vi "HandleObservationSync_003.vi"(8 "error in (no error)":errorcluster, 11 "S4GUI in":refnum<class "S4GUI.lvclass">) -> (0 "error out":errorcluster, 3 "S4GUI out":refnum<class "S4GUI.lvclass">)   [LabVIEW 2018, in "S4GUI.lvclass"] (continued)
          n1515 = call-dynamic "Write AcquisitionA.vi"("error in (no error)"=w4306, "Acquisition.lvclass"=w4308, "S4ACS_GUI in"=w4307) -> ("error out"=w4303:errorcluster, "S4ACS_GUI out"=w4302:refnum<class "S4GUI.lvclass">)  [unwired: 7 in]
          n1516 = call "Read AcquisitionB.vi"("error in (no error)"=w4303, "S4ACS_GUI in"=w4302) -> ("error out"=w4281:errorcluster, "Acquisition.lvclass"=w4284:refnum<class "Acquisition.lvclass">, "S4ACS_GUI out"=w4304:refnum<class "S4GUI.lvclass">)  [unwired: 7 in]
          n1517 = call-dynamic "Read enabled.vi"("error in (no error)"=w4281, "Server in"=w4284) -> ("error out"=w4282:errorcluster, "enabled"=w4262:bool, "Server out"=w4283:refnum<class "Acquisition.lvclass">)  [unwired: 7 in]
          n1518 = case shown="True" w4262 {
            tunnel: w4282 -> [w4437 w4454]
            tunnel: w4283 -> [w4438 w4453]
            tunnel: [0 ("State") w4446] -> w4257
            tunnel: [w4437 w4452] -> w4301
            tunnel: [w4438 w4451] -> w4300
            tunnel: w4267 -> [_ w4445]
            tunnel: [TRUE w4444] -> w4268
            tunnel: [FALSE ("stopping") w4440] -> w4253
            frame False {
            }
            frame True {
              n1519 = call-dynamic "Read Channel.vi"("error in (no error)"=w4454, "Acquisition in"=w4453) -> ("error out"=w4449:errorcluster, "Channel.lvclass"=w4450:refnum<class "Channel.lvclass">, "Acquisition out"=w4447:refnum<class "Acquisition.lvclass">)  [unwired: 7 in]
              n1520 = call-dynamic "Read CyclesDone.vi"("error in (no error)"=w4449, "Channel in"=w4450) -> ("error out"=w4442:errorcluster, "CyclesDone"=w4446:u32, "Channel out"=w4448:refnum<class "Channel.lvclass">)  [unwired: 7 in]
              n1521 = Increment(x=w4445) -> (x+1=w4439:u32)
              n1522 = Equal?(x=w4446, y=w4439) -> (x = y?=w4444:bool)
              n1523 = call-dynamic "Read stopping.vi"("error in (no error)"=w4442, "Channel in"=w4448) -> ("error out"=w4441:errorcluster, "stopping"=w4440:bool, "Channel out"=w4443:refnum<class "Channel.lvclass">)  [unwired: 7 in]
              n1524 = call-dynamic "Write Channel.vi"("error in (no error)"=w4441, "Channel.lvclass"=w4443, "Acquisition in"=w4447) -> ("error out"=w4452:errorcluster, "Acquisition out"=w4451:refnum<class "Acquisition.lvclass">)  [unwired: 7 in]
            }
          }
          n1525 = Max & Min(x=w4258, y=w4257) -> (max(x,y)=w4270:u32)  [unwired: 1 out]
          n1526 = call "Write AcquisitionB.vi"("error in (no error)"=w4301, "Acquisition.lvclass"=w4300, "S4ACS_GUI in"=w4304) -> ("error out"=w4293:errorcluster, "S4ACS_GUI out"=w4292:refnum<class "S4GUI.lvclass">)  [unwired: 7 in]
          n1527 = call-dynamic "Read AcquisitionC.vi"("error in (no error)"=w4293, "S4ACS_GUI in"=w4292) -> ("error out"=w4278:errorcluster, "Acquisition.lvclass"=w4280:refnum<class "Acquisition.lvclass">, "S4ACS_GUI out"=w4295:refnum<class "S4GUI.lvclass">)  [unwired: 7 in]
          n1528 = call-dynamic "Read enabled.vi"("error in (no error)"=w4278, "Server in"=w4280) -> ("error out"=w4277:errorcluster, "enabled"=w4261:bool, "Server out"=w4279:refnum<class "Acquisition.lvclass">)  [unwired: 7 in]
          n1529 = case shown="True" w4261 {
            tunnel: [w4416 w4433] -> w4296
            tunnel: [w4417 w4432] -> w4294
            tunnel: w4277 -> [w4416 w4429]
            tunnel: w4279 -> [w4417 w4430]
            tunnel: [0 ("State") w4428] -> w4256
            tunnel: w4267 -> [_ w4427]
            tunnel: [TRUE w4426] -> w4266
            tunnel: [FALSE ("stopping") w4419] -> w4252
            frame False {
            }
            frame True {
              n1530 = call-dynamic "Read Channel.vi"("error in (no error)"=w4429, "Acquisition in"=w4430) -> ("error out"=w4425:errorcluster, "Channel.lvclass"=w4424:refnum<class "Channel.lvclass">, "Acquisition out"=w4431:refnum<class "Acquisition.lvclass">)  [unwired: 7 in]
              n1531 = call-dynamic "Read CyclesDone.vi"("error in (no error)"=w4425, "Channel in"=w4424) -> ("error out"=w4421:errorcluster, "CyclesDone"=w4428:u32, "Channel out"=w4423:refnum<class "Channel.lvclass">)  [unwired: 7 in]
              n1532 = Increment(x=w4427) -> (x+1=w4418:u32)
              n1533 = Equal?(x=w4428, y=w4418) -> (x = y?=w4426:bool)
              n1534 = call-dynamic "Read stopping.vi"("error in (no error)"=w4421, "Channel in"=w4423) -> ("error out"=w4420:errorcluster, "stopping"=w4419:bool, "Channel out"=w4422:refnum<class "Channel.lvclass">)  [unwired: 7 in]
              n1535 = call-dynamic "Write Channel.vi"("error in (no error)"=w4420, "Channel.lvclass"=w4422, "Acquisition in"=w4431) -> ("error out"=w4433:errorcluster, "Acquisition out"=w4432:refnum<class "Acquisition.lvclass">)  [unwired: 7 in]
            }
          }
          n1536 = call-dynamic "Write AcquisitionC.vi"("error in (no error)"=w4296, "Acquisition.lvclass"=w4294, "S4ACS_GUI in"=w4295) -> ("error out"=w4290:errorcluster, "S4ACS_GUI out"=w4291:refnum<class "S4GUI.lvclass">)  [unwired: 7 in]
          n1537 = call-dynamic "Read AcquisitionD.vi"("error in (no error)"=w4290, "S4ACS_GUI in"=w4291) -> ("error out"=w4274:errorcluster, "Acquisition.lvclass"=w4276:refnum<class "Acquisition.lvclass">, "S4ACS_GUI out"=w4297:refnum<class "S4GUI.lvclass">)  [unwired: 7 in]
          n1538 = call-dynamic "Read enabled.vi"("error in (no error)"=w4274, "Server in"=w4276) -> ("error out"=w4273:errorcluster, "enabled"=w4264:bool, "Server out"=w4275:refnum<class "Acquisition.lvclass">)  [unwired: 7 in]
          n1539 = case shown="True" w4264 {
            tunnel: [w4396 w4412] -> w4299
            tunnel: [w4395 w4411] -> w4298
            tunnel: w4275 -> [w4396 w4410]
            tunnel: w4273 -> [w4395 w4409]
            tunnel: [0 ("State") w4407] -> w4255
            tunnel: w4267 -> [_ w4406]
            tunnel: [TRUE w4405] -> w4265
            tunnel: [FALSE ("stopping") w4398] -> w4251
            frame False {
            }
            frame True {
              n1540 = call-dynamic "Read Channel.vi"("error in (no error)"=w4409, "Acquisition in"=w4410) -> ("error out"=w4404:errorcluster, "Channel.lvclass"=w4403:refnum<class "Channel.lvclass">, "Acquisition out"=w4408:refnum<class "Acquisition.lvclass">)  [unwired: 7 in]
              n1541 = call-dynamic "Read CyclesDone.vi"("error in (no error)"=w4404, "Channel in"=w4403) -> ("error out"=w4400:errorcluster, "CyclesDone"=w4407:u32, "Channel out"=w4402:refnum<class "Channel.lvclass">)  [unwired: 7 in]
              n1542 = Increment(x=w4406) -> (x+1=w4397:u32)
              n1543 = Equal?(x=w4407, y=w4397) -> (x = y?=w4405:bool)
              n1544 = call-dynamic "Read stopping.vi"("error in (no error)"=w4400, "Channel in"=w4402) -> ("error out"=w4399:errorcluster, "stopping"=w4398:bool, "Channel out"=w4401:refnum<class "Channel.lvclass">)  [unwired: 7 in]
              n1545 = call-dynamic "Write Channel.vi"("error in (no error)"=w4399, "Channel.lvclass"=w4401, "Acquisition in"=w4408) -> ("error out"=w4411:errorcluster, "Acquisition out"=w4412:refnum<class "Acquisition.lvclass">)  [unwired: 7 in]
            }
          }
          n1546 = Build Array(w4263, w4262, w4261, w4264) -> (w4260:bool[])
          n1547 = Boolean Array To Number(Boolean array=w4260) -> (number=w4259:u32)
          n1548 = Max & Min(x=w4256, y=w4255) -> (max(x,y)=w4269:u32)  [unwired: 1 out]
          n1549 = Compound Arithmetic op=AND(w4271, w4268, w4266, w4265) -> (w4250:bool)
          n1550 = case shown="15" w4259 {
            tunnel: w4258 -> [w4348 _ w4360 _ w4369 _ w4375 w4381 _ w4387 w4390 _]
            tunnel: w4255 -> [w4347 w4351 w4356 w4363 w4364 w4372 w4374 _ _ _ _ _]
            tunnel: w4257 -> [w4346 w4349 _ _ w4368 w4370 _ w4380 w4384 _ w4389 _]
            tunnel: w4256 -> [w4345 w4350 w4355 w4361 _ _ _ w4379 w4383 w4386 _ _]
            tunnel: [w4341 w4352 w4357 w4362 w4365 w4371 w4373 w4376 w4382 w4385 w4388 TRUE] -> _
            frame 15 {
              # "A,B,C,D ativos"
              n1551 = Equal?(x=w4348, y=w4346) -> (x = y?=w4344:bool)
              n1552 = Equal?(x=w4345, y=w4347) -> (x = y?=w4342:bool)
              n1553 = Equal?(x=w4346, y=w4345) -> (x = y?=w4343:bool)
              n1554 = Compound Arithmetic op=AND(w4344, w4343, w4342) -> (w4341:bool)
            }
            frame 14 {
              # "B,C e,D ativos"
              n1555 = Equal?(x=w4349, y=w4350) -> (x = y?=w4354:bool)
              n1556 = Equal?(x=w4350, y=w4351) -> (x = y?=w4353:bool)
              n1557 = Compound Arithmetic op=AND(w4354, w4353) -> (w4352:bool)
            }
            frame 13 {
              # "A,C e,D ativos"
              n1558 = Equal?(x=w4360, y=w4355) -> (x = y?=w4359:bool)
              n1559 = Equal?(x=w4355, y=w4356) -> (x = y?=w4358:bool)
              n1560 = Compound Arithmetic op=AND(w4359, w4358) -> (w4357:bool)
            }
            frame 12 {
              # "Só C e D ativos"
              n1561 = Equal?(x=w4361, y=w4363) -> (x = y?=w4362:bool)
            }
            frame 11 {
              # "A,B e,D ativos"
              n1562 = Equal?(x=w4369, y=w4368) -> (x = y?=w4367:bool)
              n1563 = Equal?(x=w4368, y=w4364) -> (x = y?=w4366:bool)
              n1564 = Compound Arithmetic op=AND(w4367, w4366) -> (w4365:bool)
            }
            frame 10 {
              # "Só B e D ativos"
              n1565 = Equal?(x=w4370, y=w4372) -> (x = y?=w4371:bool)
            }
            frame 9 {
              # "Só A e D ativos"
              n1566 = Equal?(x=w4375, y=w4374) -> (x = y?=w4373:bool)
            }
            frame 7 {
              # "A,B,C ativos"
              n1567 = Equal?(x=w4381, y=w4380) -> (x = y?=w4378:bool)
              n1568 = Equal?(x=w4380, y=w4379) -> (x = y?=w4377:bool)
              n1569 = Compound Arithmetic op=AND(w4378, w4377) -> (w4376:bool)
            }
            frame 6 {
              # "Só B e C ativos"
              n1570 = Equal?(x=w4384, y=w4383) -> (x = y?=w4382:bool)
            }
            frame 5 {
              # "Só A e C ativos"
              n1571 = Equal?(x=w4387, y=w4386) -> (x = y?=w4385:bool)
            }
            frame 3 {
              # "só A e B ativos"
              n1572 = Equal?(x=w4390, y=w4389) -> (x = y?=w4388:bool)
            }
            frame 0..2, 4, 8, Default {
              # "nenhum ou só 1  \ncanal ativo."
            }
          }
          n1573 = Max & Min(x=w4270, y=w4269) -> (max(x,y)=w4248:u32)  [unwired: 1 out]
          n1574 = Compound Arithmetic op=OR(w4254, w4253, w4252, w4251) -> (w4249:bool)
          n1575 = call-dynamic "Write AcquisitionD.vi"("error in (no error)"=w4298, "Acquisition.lvclass"=w4299, "S4ACS_GUI in"=w4297) -> ("error out"=w4289:errorcluster, "S4ACS_GUI out"=w4246:refnum<class "S4GUI.lvclass">)  [unwired: 7 in]
          n1576 = case shown="False" w4250 {
            tunnel: w4246 -> [w4311 w4329]
            tunnel: [w4317 w4328] -> w4245
            tunnel: w4249 -> [_ w4330]
            tunnel: w4248 -> [_ w4327]
            tunnel: w4247 -> [w4309 w4326]
            frame False {
              # "Aguardando iniciar exposição por 5s"
              n1577 = local read "time1"() -> (w4310:u32)
              n1578 = Tick Count (ms)() -> (millisecond timer value=w4316:u32)
              n1579 = Subtract(x=w4316, y=w4310) -> (x-y=w4313:u32)
              n1580 = To Double Precision Float(number=w4313) -> (double precision float=w4315:dbl)
              n1581 = Less?(x=5000.0 ("y"), y=w4315) -> (x < y?=w4314:bool)
              n1582 = case shown="False" w4314 {
                tunnel: w4311 -> [w4321 w4325]
                tunnel: [w4320 w4324] -> w4317
                tunnel: w4309 -> [w4319 _]
                frame False {
                  # "Volta para esperar ACTIVE."
                  n1583 = Decrement(x=w4319) -> (x-1=w4318:u32)
                  n1584 = Bundle By Name(cluster=w4321, "Obs_state"=w4318) -> (w4320:refnum<class "S4GUI.lvclass">)
                }
                frame True {
                  n1585 = Bundle By Name(cluster=w4325, "Obs_state"=u32 1, "Error Msg"="ERROR: Init Acquisition Timeout. HandleObservationSync.vi - state 327.") -> (w4324:refnum<class "S4GUI.lvclass">)
                }
              }
            }
            frame True {
              # "STOP?"
              # "CIclo Avançou."
              n1586 = case shown="False" w4330 {
                tunnel: w4329 -> [w4334 w4340]
                tunnel: [w4333 w4339] -> w4328
                tunnel: w4327 -> [w4332 w4338]
                tunnel: w4326 -> [_ w4337]
                frame True {
                  # "STOP acionado."
                  n1587 = Bundle By Name(cluster=w4334, "Obs_state"=u32 0, "cyclesDone"=w4332) -> (w4333:refnum<class "S4GUI.lvclass">)
                }
                frame False {
                  # "Vai esperar fim da exposição..."
                  n1588 = Increment(x=w4337) -> (x+1=w4336:u32)
                  n1589 = Increment(x=w4336) -> (x+1=w4335:u32)
                  n1590 = Bundle By Name(cluster=w4340, "Obs_state"=w4335, "cyclesDone"=w4338) -> (w4339:refnum<class "S4GUI.lvclass">)
                }
              }
            }
          }
        }
        frame 328 {
          # "T= canais receberam STOP"
          n1591 = Unbundle By Name(w4500) -> ("cyclesDone"=w4494:u32)
          n1592 = call-dynamic "Read AcquisitionA.vi"("error in (no error)"=w4536, "S4ACS_GUI in"=w4500) -> ("error out"=w4515:errorcluster, "Acquisition.lvclass"=w4516:refnum<class "Acquisition.lvclass">, "S4ACS_GUI out"=w4538:refnum<class "S4GUI.lvclass">)  [unwired: 7 in]
          n1593 = call-dynamic "Read enabled.vi"("error in (no error)"=w4515, "Server in"=w4516) -> ("error out"=w4514:errorcluster, "enabled"=w4490:bool, "Server out"=w4513:refnum<class "Acquisition.lvclass">)  [unwired: 7 in]
          n1594 = case shown="True" w4490 {
            tunnel: w4514 -> [w4687 w4704]
            tunnel: [w4688 w4702] -> w4539
            tunnel: [w4687 w4701] -> w4537
            tunnel: [0 ("State") w4697] -> w4485
            tunnel: w4513 -> [w4688 w4696]
            tunnel: w4494 -> [_ w4695]
            tunnel: [TRUE w4694] -> w4499
            tunnel: [FALSE ("stopping") w4690] -> w4481
            frame False {
            }
            frame True {
              n1595 = call-dynamic "Read Channel.vi"("error in (no error)"=w4704, "Acquisition in"=w4696) -> ("error out"=w4700:errorcluster, "Channel.lvclass"=w4699:refnum<class "Channel.lvclass">, "Acquisition out"=w4703:refnum<class "Acquisition.lvclass">)  [unwired: 7 in]
              n1596 = call-dynamic "Read CyclesDone.vi"("error in (no error)"=w4700, "Channel in"=w4699) -> ("error out"=w4692:errorcluster, "CyclesDone"=w4697:u32, "Channel out"=w4698:refnum<class "Channel.lvclass">)  [unwired: 7 in]
              n1597 = Increment(x=w4695) -> (x+1=w4689:u32)
              n1598 = Equal?(x=w4697, y=w4689) -> (x = y?=w4694:bool)
              n1599 = call-dynamic "Read stopping.vi"("error in (no error)"=w4692, "Channel in"=w4698) -> ("error out"=w4691:errorcluster, "stopping"=w4690:bool, "Channel out"=w4693:refnum<class "Channel.lvclass">)  [unwired: 7 in]
              n1600 = call-dynamic "Write Channel.vi"("error in (no error)"=w4691, "Channel.lvclass"=w4693, "Acquisition in"=w4703) -> ("error out"=w4701:errorcluster, "Acquisition out"=w4702:refnum<class "Acquisition.lvclass">)  [unwired: 7 in]
            }
          }
          n1601 = call-dynamic "Write AcquisitionA.vi"("error in (no error)"=w4537, "Acquisition.lvclass"=w4539, "S4ACS_GUI in"=w4538) -> ("error out"=w4532:errorcluster, "S4ACS_GUI out"=w4531:refnum<class "S4GUI.lvclass">)  [unwired: 7 in]
          n1602 = call "Read AcquisitionB.vi"("error in (no error)"=w4532, "S4ACS_GUI in"=w4531) -> ("error out"=w4509:errorcluster, "Acquisition.lvclass"=w4512:refnum<class "Acquisition.lvclass">, "S4ACS_GUI out"=w4533:refnum<class "S4GUI.lvclass">)  [unwired: 7 in]
          n1603 = call-dynamic "Read enabled.vi"("error in (no error)"=w4509, "Server in"=w4512) -> ("error out"=w4510:errorcluster, "enabled"=w4489:bool, "Server out"=w4511:refnum<class "Acquisition.lvclass">)  [unwired: 7 in]
          n1604 = case shown="True" w4489 {
            tunnel: w4510 -> [w4666 w4683]
            tunnel: w4511 -> [w4667 w4682]
            tunnel: [0 ("State") w4675] -> w4484
            tunnel: [w4666 w4681] -> w4530
            tunnel: [w4667 w4680] -> w4529
            tunnel: w4494 -> [_ w4674]
            tunnel: [TRUE w4673] -> w4495
            tunnel: [FALSE ("stopping") w4669] -> w4480
            frame False {
            }
            frame True {
              n1605 = call-dynamic "Read Channel.vi"("error in (no error)"=w4683, "Acquisition in"=w4682) -> ("error out"=w4678:errorcluster, "Channel.lvclass"=w4679:refnum<class "Channel.lvclass">, "Acquisition out"=w4676:refnum<class "Acquisition.lvclass">)  [unwired: 7 in]
              n1606 = call-dynamic "Read CyclesDone.vi"("error in (no error)"=w4678, "Channel in"=w4679) -> ("error out"=w4671:errorcluster, "CyclesDone"=w4675:u32, "Channel out"=w4677:refnum<class "Channel.lvclass">)  [unwired: 7 in]
              n1607 = Increment(x=w4674) -> (x+1=w4668:u32)
              n1608 = Equal?(x=w4675, y=w4668) -> (x = y?=w4673:bool)
              n1609 = call-dynamic "Read stopping.vi"("error in (no error)"=w4671, "Channel in"=w4677) -> ("error out"=w4670:errorcluster, "stopping"=w4669:bool, "Channel out"=w4672:refnum<class "Channel.lvclass">)  [unwired: 7 in]
              n1610 = call-dynamic "Write Channel.vi"("error in (no error)"=w4670, "Channel.lvclass"=w4672, "Acquisition in"=w4676) -> ("error out"=w4681:errorcluster, "Acquisition out"=w4680:refnum<class "Acquisition.lvclass">)  [unwired: 7 in]
            }
          }
          n1611 = Max & Min(x=w4485, y=w4484) -> (max(x,y)=w4498:u32)  [unwired: 1 out]
          n1612 = call "Write AcquisitionB.vi"("error in (no error)"=w4530, "Acquisition.lvclass"=w4529, "S4ACS_GUI in"=w4533) -> ("error out"=w4522:errorcluster, "S4ACS_GUI out"=w4521:refnum<class "S4GUI.lvclass">)  [unwired: 7 in]
          n1613 = call-dynamic "Read AcquisitionC.vi"("error in (no error)"=w4522, "S4ACS_GUI in"=w4521) -> ("error out"=w4506:errorcluster, "Acquisition.lvclass"=w4508:refnum<class "Acquisition.lvclass">, "S4ACS_GUI out"=w4524:refnum<class "S4GUI.lvclass">)  [unwired: 7 in]
          n1614 = call-dynamic "Read enabled.vi"("error in (no error)"=w4506, "Server in"=w4508) -> ("error out"=w4505:errorcluster, "enabled"=w4488:bool, "Server out"=w4507:refnum<class "Acquisition.lvclass">)  [unwired: 7 in]
          n1615 = case shown="True" w4488 {
            tunnel: [w4645 w4662] -> w4525
            tunnel: [w4646 w4661] -> w4523
            tunnel: w4505 -> [w4645 w4658]
            tunnel: w4507 -> [w4646 w4659]
            tunnel: [0 ("State") w4657] -> w4483
            tunnel: w4494 -> [_ w4656]
            tunnel: [TRUE w4655] -> w4493
            tunnel: [FALSE ("stopping") w4648] -> w4479
            frame False {
            }
            frame True {
              n1616 = call-dynamic "Read Channel.vi"("error in (no error)"=w4658, "Acquisition in"=w4659) -> ("error out"=w4654:errorcluster, "Channel.lvclass"=w4653:refnum<class "Channel.lvclass">, "Acquisition out"=w4660:refnum<class "Acquisition.lvclass">)  [unwired: 7 in]
              n1617 = call-dynamic "Read CyclesDone.vi"("error in (no error)"=w4654, "Channel in"=w4653) -> ("error out"=w4650:errorcluster, "CyclesDone"=w4657:u32, "Channel out"=w4652:refnum<class "Channel.lvclass">)  [unwired: 7 in]
              n1618 = Increment(x=w4656) -> (x+1=w4647:u32)
              n1619 = Equal?(x=w4657, y=w4647) -> (x = y?=w4655:bool)
              n1620 = call-dynamic "Read stopping.vi"("error in (no error)"=w4650, "Channel in"=w4652) -> ("error out"=w4649:errorcluster, "stopping"=w4648:bool, "Channel out"=w4651:refnum<class "Channel.lvclass">)  [unwired: 7 in]
              n1621 = call-dynamic "Write Channel.vi"("error in (no error)"=w4649, "Channel.lvclass"=w4651, "Acquisition in"=w4660) -> ("error out"=w4662:errorcluster, "Acquisition out"=w4661:refnum<class "Acquisition.lvclass">)  [unwired: 7 in]
            }
          }
          n1622 = call-dynamic "Write AcquisitionC.vi"("error in (no error)"=w4525, "Acquisition.lvclass"=w4523, "S4ACS_GUI in"=w4524) -> ("error out"=w4519:errorcluster, "S4ACS_GUI out"=w4520:refnum<class "S4GUI.lvclass">)  [unwired: 7 in]
          n1623 = call-dynamic "Read AcquisitionD.vi"("error in (no error)"=w4519, "S4ACS_GUI in"=w4520) -> ("error out"=w4502:errorcluster, "Acquisition.lvclass"=w4504:refnum<class "Acquisition.lvclass">, "S4ACS_GUI out"=w4526:refnum<class "S4GUI.lvclass">)  [unwired: 7 in]
          n1624 = call-dynamic "Read enabled.vi"("error in (no error)"=w4502, "Server in"=w4504) -> ("error out"=w4501:errorcluster, "enabled"=w4491:bool, "Server out"=w4503:refnum<class "Acquisition.lvclass">)  [unwired: 7 in]
          n1625 = case shown="True" w4491 {
            tunnel: [w4625 w4641] -> w4528
            tunnel: [w4624 w4640] -> w4527
            tunnel: w4503 -> [w4625 w4639]
            tunnel: w4501 -> [w4624 w4638]
            tunnel: [0 ("State") w4636] -> w4482
            tunnel: w4494 -> [_ w4635]
            tunnel: [TRUE w4634] -> w4492
            tunnel: [FALSE ("stopping") w4627] -> w4478
            frame False {
            }
            frame True {
              n1626 = call-dynamic "Read Channel.vi"("error in (no error)"=w4638, "Acquisition in"=w4639) -> ("error out"=w4633:errorcluster, "Channel.lvclass"=w4632:refnum<class "Channel.lvclass">, "Acquisition out"=w4637:refnum<class "Acquisition.lvclass">)  [unwired: 7 in]
              n1627 = call-dynamic "Read CyclesDone.vi"("error in (no error)"=w4633, "Channel in"=w4632) -> ("error out"=w4629:errorcluster, "CyclesDone"=w4636:u32, "Channel out"=w4631:refnum<class "Channel.lvclass">)  [unwired: 7 in]
              n1628 = Increment(x=w4635) -> (x+1=w4626:u32)
              n1629 = Equal?(x=w4636, y=w4626) -> (x = y?=w4634:bool)
              n1630 = call-dynamic "Read stopping.vi"("error in (no error)"=w4629, "Channel in"=w4631) -> ("error out"=w4628:errorcluster, "stopping"=w4627:bool, "Channel out"=w4630:refnum<class "Channel.lvclass">)  [unwired: 7 in]
              n1631 = call-dynamic "Write Channel.vi"("error in (no error)"=w4628, "Channel.lvclass"=w4630, "Acquisition in"=w4637) -> ("error out"=w4640:errorcluster, "Acquisition out"=w4641:refnum<class "Acquisition.lvclass">)  [unwired: 7 in]
            }
          }
          n1632 = Build Array(w4490, w4489, w4488, w4491) -> (w4487:bool[])
          n1633 = Boolean Array To Number(Boolean array=w4487) -> (number=w4486:u32)
          n1634 = Max & Min(x=w4483, y=w4482) -> (max(x,y)=w4497:u32)  [unwired: 1 out]
          n1635 = Compound Arithmetic op=AND(w4499, w4495, w4493, w4492) -> (w4476:bool)
          n1636 = case shown="15" w4486 {
            tunnel: w4485 -> [w4547 _ w4559 _ w4568 _ w4574 w4580 _ w4586 w4589 _]
            tunnel: w4482 -> [w4546 w4550 w4555 w4562 w4563 w4571 w4573 _ _ _ _ _]
            tunnel: w4484 -> [w4545 w4548 _ _ w4567 w4569 _ w4579 w4583 _ w4588 _]
            tunnel: w4483 -> [w4544 w4549 w4554 w4560 _ _ _ w4578 w4582 w4585 _ _]
            tunnel: [w4540 w4551 w4556 w4561 w4564 w4570 w4572 w4575 w4581 w4584 w4587 TRUE] -> _
            frame 15 {
              # "A,B,C,D ativos"
              n1637 = Equal?(x=w4547, y=w4545) -> (x = y?=w4543:bool)
              n1638 = Equal?(x=w4544, y=w4546) -> (x = y?=w4541:bool)
              n1639 = Equal?(x=w4545, y=w4544) -> (x = y?=w4542:bool)
              n1640 = Compound Arithmetic op=AND(w4543, w4542, w4541) -> (w4540:bool)
            }
            frame 14 {
              # "B,C e,D ativos"
              n1641 = Equal?(x=w4548, y=w4549) -> (x = y?=w4553:bool)
              n1642 = Equal?(x=w4549, y=w4550) -> (x = y?=w4552:bool)
              n1643 = Compound Arithmetic op=AND(w4553, w4552) -> (w4551:bool)
            }
            frame 13 {
              # "A,C e,D ativos"
              n1644 = Equal?(x=w4559, y=w4554) -> (x = y?=w4558:bool)
              n1645 = Equal?(x=w4554, y=w4555) -> (x = y?=w4557:bool)
              n1646 = Compound Arithmetic op=AND(w4558, w4557) -> (w4556:bool)
            }
            frame 12 {
              # "Só C e D ativos"
              n1647 = Equal?(x=w4560, y=w4562) -> (x = y?=w4561:bool)
            }
            frame 11 {
              # "A,B e,D ativos"
              n1648 = Equal?(x=w4568, y=w4567) -> (x = y?=w4566:bool)
              n1649 = Equal?(x=w4567, y=w4563) -> (x = y?=w4565:bool)
              n1650 = Compound Arithmetic op=AND(w4566, w4565) -> (w4564:bool)
            }
            frame 10 {
              # "Só B e D ativos"
              n1651 = Equal?(x=w4569, y=w4571) -> (x = y?=w4570:bool)
            }
            frame 9 {
              # "Só A e D ativos"
              n1652 = Equal?(x=w4574, y=w4573) -> (x = y?=w4572:bool)
            }
            frame 7 {
              # "A,B,C ativos"
              n1653 = Equal?(x=w4580, y=w4579) -> (x = y?=w4577:bool)
              n1654 = Equal?(x=w4579, y=w4578) -> (x = y?=w4576:bool)
              n1655 = Compound Arithmetic op=AND(w4577, w4576) -> (w4575:bool)
            }
            frame 6 {
              # "Só B e C ativos"
              n1656 = Equal?(x=w4583, y=w4582) -> (x = y?=w4581:bool)
            }
            frame 5 {
              # "Só A e C ativos"
              n1657 = Equal?(x=w4586, y=w4585) -> (x = y?=w4584:bool)
            }
            frame 3 {
              # "só A e B ativos"
              n1658 = Equal?(x=w4589, y=w4588) -> (x = y?=w4587:bool)
            }
            frame 0..2, 4, 8, Default {
              # "nenhum ou só 1  \ncanal ativo."
            }
          }
          n1659 = Max & Min(x=w4498, y=w4497) -> (max(x,y)=w4496:u32)  [unwired: 1 out]
          n1660 = Compound Arithmetic op=OR(w4481, w4480, w4479, w4478) -> (w4477:bool)
          n1661 = call-dynamic "Write AcquisitionD.vi"("error in (no error)"=w4527, "Acquisition.lvclass"=w4528, "S4ACS_GUI in"=w4526) -> ("error out"=w4517:errorcluster, "S4ACS_GUI out"=w4518:refnum<class "S4GUI.lvclass">)  [unwired: 7 in]
          n1662 = case shown="True" w4476 {
            tunnel: w4518 -> [w4601 w4611]
            tunnel: [w4600 w4610] -> w4535
            tunnel: w4534 -> [_ w4609]
            tunnel: w4496 -> [_ w4608]
            tunnel: w4477 -> [_ w4607]
            frame False {
              # "Aguardando avanço do ciclo."
              n1663 = local read "time307"() -> (w4591:u32)
              n1664 = Tick Count (ms)() -> (millisecond timer value=w4599:u32)
              n1665 = Subtract(x=w4599, y=w4591) -> (x-y=w4596:u32)
              n1666 = call-dynamic "GetGreatestCube.vi"("S4GUI in"=w4601) -> ("S4GUI out"=w4592:refnum<class "S4GUI.lvclass">, "greatest (ms)"=w4594:dbl)  [unwired: 8 in, 1 out]
              n1667 = To Double Precision Float(number=w4596) -> (double precision float=w4598:dbl)
              n1668 = Add(x=5000.0 ("y"), y=w4594) -> (x+y=w4593:dbl)
              n1669 = Less?(x=w4593, y=w4598) -> (x < y?=w4597:bool)
              n1670 = case shown="True" w4597 {
                tunnel: w4592 -> [w4602 w4606]
                tunnel: [w4602 w4605] -> w4600
                frame False {
                }
                frame True {
                  n1671 = Bundle By Name(cluster=w4606, "Obs_state"=u32 1, "Error Msg"="ERROR: Acquisition Timeout. HandleObservationSync.vi - state 328.") -> (w4605:refnum<class "S4GUI.lvclass">)
                }
              }
            }
            frame True {
              # "Ciclo avançou."
              # "STOP?"
              n1672 = case shown="False" w4607 {
                tunnel: w4611 -> [w4615 w4620]
                tunnel: [w4614 w4619] -> w4610
                tunnel: w4609 -> [_ w4617]
                tunnel: w4608 -> [w4613 w4616]
                frame True {
                  n1673 = Bundle By Name(cluster=w4615, "Obs_state"=u32 0, "cyclesDone"=w4613) -> (w4614:refnum<class "S4GUI.lvclass">)
                }
                frame False {
                  n1674 = Increment(x=w4617) -> (x+1=w4618:u32)
                  n1675 = Bundle By Name(cluster=w4620, "Obs_state"=w4618, "cyclesDone"=w4616) -> (w4619:refnum<class "S4GUI.lvclass">)
                }
              }
            }
          }
        }
        frame 329 {
          n1676 = disable-structure shown="Enabled" {
            disable-tunnel: w4709 -> [w4723 w4729]
            disable-tunnel: w4708 -> [w4722 w4736]
            disable-tunnel: [w4721 w4736] -> w4707
            disable-tunnel: [w4719 w4737] -> w4706
            disable-tunnel: w4705 -> [_ w4730]
            frame Disabled {
              n1677 = call-dynamic "Read ciclos.vi"("error in (no error)"=w4722, "S4ACS_GUI in"=w4723) -> ("error out"=w4711:errorcluster, "ciclos"=w4716:u32, "S4ACS_GUI out"=w4724:refnum<class "S4GUI.lvclass">)  [unwired: 7 in]
              n1678 = Decrement(x=w4716) -> (x-1=w4710:u32)
              n1679 = Greater Than 0?(x=w4710) -> (x > 0?=w4717:bool)
              n1680 = case shown="False" w4717 {
                selector: w4717 -> [w4726 w4728]
                tunnel: w4710 -> [_ w4727]
                tunnel: [w4726 w4728] -> w4715
                tunnel: [u32 0 w4727] -> w4712
                frame False {
                }
                frame True {
                }
              }
              n1681 = Select(t=u32 323, s=w4715, f=u32 0) -> (s? t:f=w4718:u32)
              n1682 = call-dynamic "Write ciclos.vi"("error in (no error)"=w4711, "ciclos"=w4712, "S4ACS_GUI in"=w4724) -> ("error out"=w4721:errorcluster, "S4ACS_GUI out"=w4720:refnum<class "S4GUI.lvclass">)  [unwired: 7 in]
              n1683 = Bundle By Name(cluster=w4720, "Obs_state"=w4718) -> (w4719:refnum<class "S4GUI.lvclass">)
            }
            frame Enabled {
              n1684 = Unbundle By Name(w4729) -> ("TotalCiclos"=w4739:u32, "cyclesDone"=w4738:u32)
              n1685 = Subtract(x=w4739, y=w4738) -> (x-y=w4732:u32)
              n1686 = Greater Than 0?(x=w4732) -> (x > 0?=w4735:bool)
              n1687 = disable-structure shown="Enabled" {
                disable-tunnel: [w4741 u32 325 ("t")] -> w4731
                disable-tunnel: w4730 -> [w4740 _]
                frame Disabled {
                  n1688 = Increment(x=w4740) -> (x+1=w4741:u32)
                }
                frame Enabled {
                }
              }
              n1689 = Select(t=w4731, s=w4735, f=u32 0) -> (s? t:f=w4734:u32)
              n1690 = Bundle By Name(cluster=w4729, "ciclos"=w4732, "Obs_state"=w4734) -> (w4737:refnum<class "S4GUI.lvclass">)
            }
          }
        }
        frame 350 {
          n1691 = flat-sequence {
            tunnel: w4744 -> [w4784]
            tunnel: [w4784] -> w4743
            frame #0 {
              n1692 = Tick Count (ms)() -> (millisecond timer value=→"timer350":u32)
            }
          }
          n1693 = call "Read Instrument.lvclass.vi"("error in (no error)"=w4743, "S4ACS_GUI in"=w4779) -> ("error out"=w4782:errorcluster, "Instrument.lvclass"=w4783:refnum<class "Instrument.lvclass">, "S4ACS_GUI out"=w4780:refnum<class "S4GUI.lvclass">)  [unwired: 7 in]
          n1694 = call "Read WPROT.vi"("error in (no error)"=w4782, "Instrument in"=w4783) -> ("error out"=w4772:errorcluster, "Opt_Selector.lvclass"=w4773:refnum<class "Opt_Selector.lvclass">, "Instrument out"=w4781:refnum<class "Instrument.lvclass">)  [unwired: 7 in]
          n1695 = call-dynamic "getTargetPos.vi"("error in (no error)"=w4772, "Opt_Selector in"=w4773) -> ("error out"=w4771:errorcluster, "Target Pos"=w4751:u16, "Opt_Selector out"=w4770:refnum<class "Opt_Selector.lvclass">)  [unwired: 7 in]
          n1696 = Build Array(-1.0 ("element"), 0.0 ("element"), 22.5 ("element"), 45.0 ("element"), 67.5 ("element"), 90.0 ("element"), 112.5 ("element"), 135.0 ("element"), 157.5 ("element"), 180.0 ("element"), 202.5 ("element"), 225.0 ("element"), 247.5 ("element"), 270.0 ("element"), 292.5 ("element"), 315.0 ("element"), 337.5 ("element")) -> (w4763:dbl[])
          n1697 = Index Array(array=w4763, index=w4751) -> (element=w4750:dbl)
          n1698 = case shown="0, Default" w4751 {
            selector: w4751 -> [_ w4813]
            tunnel: w4781 -> [w4793 w4801]
            tunnel: [w4793 w4801] -> w4746
            tunnel: [w4790 w4800] -> w4745
            tunnel: w4776 -> [_ w4815]
            tunnel: [u32 352 w4814] -> w4775
            tunnel: w4771 -> [w4791 w4809]
            tunnel: w4770 -> [w4792 w4808]
            tunnel: w4750 -> [_ w4803]
            tunnel: [w4788 w4802] -> w4747
            frame 0, Default {
              # "Terminou uma sequência.\nRecupera as posições em SEQ e desvia para 311 para verificar se há mais ciclos."
              # "Recupera a sequencia anterior para o caso \nde repetição da sequencia (sem precisar clicar \nnas posicoes desejadas novamente)."
              n1699 = call-dynamic "Read sequencia_ant.vi"("error in (no error)"=w4791, "Opt_Selector in"=w4792) -> ("error out"=w4787:errorcluster, "sequencia_ant"=w4786:u16, "Opt_Selector out"=w4789:refnum<class "Opt_Selector.lvclass">)  [unwired: 7 in]
              n1700 = call-dynamic "Write sequencia.vi"("error in (no error)"=w4787, "sequencia"=w4786, "Opt_Selector in"=w4789) -> ("error out"=w4790:errorcluster, "Opt_Selector out"=w4788:refnum<class "Opt_Selector.lvclass">)  [unwired: 7 in]
            }
            frame 1..16 {
              # "Espera até 40 x 0.25s (= 10s) para\nmecanismo entrar em READY"
              n1701 = Number To Decimal String(number=w4813) -> (decimal integer string=w4812:string)  [unwired: 1 in]
              n1702 = Concatenate Strings("WP" ("string"), w4812) -> (w4810:string)
              n1703 = call "Write target name.vi"("error in (no error)"=w4809, "target name"=w4810, "Optics in"=w4808) -> ("error out"=w4806:errorcluster, "Optics out"=w4807:refnum<class "Opt_Selector.lvclass">)  [unwired: 7 in]
              n1704 = call "Write target.vi"("error in (no error)"=w4806, "target"=w4803, "Optics in"=w4807) -> ("error out"=w4805:errorcluster, "Optics out"=w4804:refnum<class "Opt_Selector.lvclass">)  [unwired: 7 in]
              n1705 = call-dynamic "Read State Machine.vi"("error in (no error)"=w4805, "Device in"=w4804) -> ("error out"=w4817:errorcluster, "State Machine.lvclass"=w4819:refnum<class "State Machine.lvclass">, "Device out"=w4816:refnum<class "Opt_Selector.lvclass">)  [unwired: 7 in]
              n1706 = Increment(x=w4815) -> (x+1=w4814:u32)
              n1707 = call "Next State.vi"("error in (no error)"=w4817, "New_State"=1, "State Machine in"=w4819) -> ("error out"=w4797:errorcluster, "State Machine out"=w4799:refnum<class "State Machine.lvclass">)  [unwired: 7 in]
              n1708 = call-dynamic "Write Timer.vi"("error in (no error)"=w4797, "Timer"=u32 40, "State Machine in"=w4799) -> ("error out"=w4796:errorcluster, "State Machine out"=w4798:refnum<class "State Machine.lvclass">)  [unwired: 7 in]
              n1709 = call-dynamic "Write State Machine.vi"("error in (no error)"=w4796, "State Machine.lvclass"=w4798, "Device in"=w4816) -> ("error out"=w4800:errorcluster, "Device out"=w4802:refnum<class "Opt_Selector.lvclass">)  [unwired: 7 in]
            }
          }
          n1710 = call "Write WPROT.vi"("error in (no error)"=w4745, "Opt_Selector.lvclass"=w4747, "Instrument in"=w4746) -> ("error out"=w4749:errorcluster, "Instrument out"=w4748:refnum<class "Instrument.lvclass">)  [unwired: 7 in]
          n1711 = call "Write Instrument.lvclass.vi"("error in (no error)"=w4749, "Instrument.lvclass"=w4748, "S4ACS_GUI in"=w4780) -> ("error out"=w4778:errorcluster, "S4ACS_GUI out"=w4777:refnum<class "S4GUI.lvclass">)  [unwired: 7 in]
          n1712 = Bundle By Name(cluster=w4777, "Obs_state"=w4775) -> (w4774:refnum<class "S4GUI.lvclass">)
        }
        frame 351 {
          # "Espera terminar o movimento da lamina para disparar a aquisição\ndos canais ativos.\n\nOV 20230424: Não precisa mais atualizar o valor de WPPOS com o\ncomando WRITE_HEADER porque o ACS já recebeu a sequência de\nposições da lâmina."
          n1713 = flat-sequence {
            tunnel: w4830 -> [w4849]
            tunnel: [w4849] -> w4829
            frame #0 {
              n1714 = Tick Count (ms)() -> (millisecond timer value=w4848:u32)
              "timer351" <- w4848
              n1715 = local read "time1"() -> (w4847:u32)
              n1716 = Subtract(x=w4848, y=w4847) -> (x-y=→"delay wp 2":u32)
            }
          }
          n1717 = call "Read Instrument.lvclass.vi"("error in (no error)"=w4829, "S4ACS_GUI in"=w4839) -> ("error out"=w4844:errorcluster, "Instrument.lvclass"=w4845:refnum<class "Instrument.lvclass">, "S4ACS_GUI out"=w4841:refnum<class "S4GUI.lvclass">)  [unwired: 7 in]
          n1718 = call "Read WPROT.vi"("error in (no error)"=w4844, "Instrument in"=w4845) -> ("error out"=w4836:errorcluster, "Opt_Selector.lvclass"=w4835:refnum<class "Opt_Selector.lvclass">, "Instrument out"=w4843:refnum<class "Instrument.lvclass">)  [unwired: 7 in]
          n1719 = call-dynamic "Read State Machine.vi"("error in (no error)"=w4836, "Device in"=w4835) -> ("error out"=w4837:errorcluster, "State Machine.lvclass"=w4838:refnum<class "State Machine.lvclass">, "Device out"=w4833:refnum<class "Opt_Selector.lvclass">)  [unwired: 7 in]
          n1720 = call-dynamic "Read State.vi"("error in (no error)"=w4837, "State Machine in"=w4838) -> ("error out"=w4827:errorcluster, "State"=w4831:i32, "State Machine out"=w4828:refnum<class "State Machine.lvclass">)  [unwired: 7 in]
          n1721 = Equal To 0?(x=w4831) -> (x = 0?=w4822:bool)
          n1722 = call-dynamic "Write State Machine.vi"("error in (no error)"=w4827, "State Machine.lvclass"=w4828, "Device in"=w4833) -> ("error out"=w4832:errorcluster, "Device out"=w4834:refnum<class "Opt_Selector.lvclass">)  [unwired: 7 in]
          n1723 = call "Write WPROT.vi"("error in (no error)"=w4832, "Opt_Selector.lvclass"=w4834, "Instrument in"=w4843) -> ("error out"=w4840:errorcluster, "Instrument out"=w4842:refnum<class "Instrument.lvclass">)  [unwired: 7 in]
          n1724 = call "Write Instrument.lvclass.vi"("error in (no error)"=w4840, "Instrument.lvclass"=w4842, "S4ACS_GUI in"=w4841) -> ("error out"=w4820:errorcluster, "S4ACS_GUI out"=w4823:refnum<class "S4GUI.lvclass">)  [unwired: 7 in]
          n1725 = Select(t=u32 350, s=w4822, f=w4821) -> (s? t:f=w4826:u32)
          n1726 = Bundle By Name(cluster=w4823, "Obs_state"=w4826) -> (w4824:refnum<class "S4GUI.lvclass">)
        }
        frame 352 {
          n1727 = disable-structure shown="Enabled" {
            disable-tunnel: w4853 -> [w4867 w4880]
            disable-tunnel: w4852 -> [w4866 w4878]
            disable-tunnel: [w4865 w4878] -> w4851
            disable-tunnel: [w4863 w4879] -> w4850
            frame Disabled {
              n1728 = call-dynamic "Read ciclos.vi"("error in (no error)"=w4866, "S4ACS_GUI in"=w4867) -> ("error out"=w4855:errorcluster, "ciclos"=w4860:u32, "S4ACS_GUI out"=w4868:refnum<class "S4GUI.lvclass">)  [unwired: 7 in]
              n1729 = Decrement(x=w4860) -> (x-1=w4854:u32)
              n1730 = Greater Than 0?(x=w4854) -> (x > 0?=w4861:bool)
              n1731 = case shown="False" w4861 {
                selector: w4861 -> [w4870 w4872]
                tunnel: w4854 -> [_ w4871]
                tunnel: [w4870 w4872] -> w4859
                tunnel: [u32 0 w4871] -> w4856
                frame False {
                }
                frame True {
                }
              }
              n1732 = Select(t=u32 323, s=w4859, f=u32 0) -> (s? t:f=w4862:u32)
              n1733 = call-dynamic "Write ciclos.vi"("error in (no error)"=w4855, "ciclos"=w4856, "S4ACS_GUI in"=w4868) -> ("error out"=w4865:errorcluster, "S4ACS_GUI out"=w4864:refnum<class "S4GUI.lvclass">)  [unwired: 7 in]
              n1734 = Bundle By Name(cluster=w4864, "Obs_state"=w4862) -> (w4863:refnum<class "S4GUI.lvclass">)
            }
            frame Enabled {
              n1735 = Unbundle By Name(w4880) -> ("cycles wprot"=w4881:u32)
              n1736 = Decrement(x=w4881) -> (x-1=w4873:u32)
              n1737 = Greater Than 0?(x=w4873) -> (x > 0?=w4877:bool)
              n1738 = Select(t=u32 350, s=w4877, f=u32 0) -> (s? t:f=w4876:u32)
              n1739 = Bundle By Name(cluster=w4880, "Obs_state"=w4876, "cycles wprot"=w4873) -> (w4879:refnum<class "S4GUI.lvclass">)
            }
          }
        }
        frame 360 {
          w4882 = u32 0 ("cyclesDone")
          # "Inicia o Ticks com\nvalor do relogio atual"
          # "Espera até 40 x 0.25s (= 10s) para\nmecanismo entrar em READY"
          # "Busca próximo valor de foco..."
          n1740 = flat-sequence {
            tunnel: w4899 -> [w4914]
            tunnel: [w4914] -> w4898
            frame #0 {
              n1741 = Tick Count (ms)() -> (millisecond timer value=→"time7":u32)
            }
          }
          n1742 = call-dynamic "Read TelFocus.lvclass.vi"("error in (no error)"=w4898, "S4GUI in"=w4910) -> ("error out"=w4912:errorcluster, "TelFocus.lvclass"=w4913:refnum<class "TelFocus.lvclass">, "S4GUI out"=w4911:refnum<class "S4GUI.lvclass">)  [unwired: 7 in]
          n1743 = call-dynamic "GetNextFocus.vi"("error in (no error)"=w4912, "TelFocus in"=w4913) -> ("error out"=w4896:errorcluster, "TelFocus out"=w4897:refnum<class "TelFocus.lvclass">)  [unwired: 8 in]
          n1744 = call-dynamic "Read SecMirror.lvclass.vi"("error in (no error)"=w4896, "TelFocus in"=w4897) -> ("error out"=w4883:errorcluster, "SecMirror.lvclass"=w4884:refnum<class "SecMirror.lvclass">, "TelFocus out"=w4901:refnum<class "TelFocus.lvclass">)  [unwired: 7 in]
          n1745 = call-dynamic "Read State Machine.vi"("error in (no error)"=w4883, "Device in"=w4884) -> ("error out"=w4893:errorcluster, "State Machine.lvclass"=w4895:refnum<class "State Machine.lvclass">, "Device out"=w4892:refnum<class "SecMirror.lvclass">)  [unwired: 7 in]
          n1746 = call "Next State.vi"("error in (no error)"=w4893, "New_State"=1, "State Machine in"=w4895) -> ("error out"=w4890:errorcluster, "State Machine out"=w4891:refnum<class "State Machine.lvclass">)  [unwired: 7 in]
          n1747 = call-dynamic "Write Timer.vi"("error in (no error)"=w4890, "Timer"=u32 40, "State Machine in"=w4891) -> ("error out"=w4887:errorcluster, "State Machine out"=w4888:refnum<class "State Machine.lvclass">)  [unwired: 7 in]
          n1748 = call-dynamic "Init Ticks2.vi"("error in (no error)"=w4887, "State Machine in"=w4888) -> ("error out"=w4886:errorcluster, "State Machine out"=w4885:refnum<class "State Machine.lvclass">)  [unwired: 8 in]
          n1749 = call-dynamic "Write State Machine.vi"("error in (no error)"=w4886, "State Machine.lvclass"=w4885, "Device in"=w4892) -> ("error out"=w4900:errorcluster, "Device out"=w4902:refnum<class "SecMirror.lvclass">)  [unwired: 7 in]
          n1750 = call-dynamic "Write SecMirror.lvclass.vi"("error in (no error)"=w4900, "SecMirror.lvclass"=w4902, "TelFocus in"=w4901) -> ("error out"=w4904:errorcluster, "TelFocus out"=w4903:refnum<class "TelFocus.lvclass">)  [unwired: 7 in]
          n1751 = call-dynamic "Write TelFocus.lvclass.vi"("error in (no error)"=w4904, "TelFocus.lvclass"=w4903, "S4GUI in"=w4911) -> ("error out"=w4909:errorcluster, "S4GUI out"=w4908:refnum<class "S4GUI.lvclass">)  [unwired: 7 in]
          n1752 = Increment(x=w4907) -> (x+1=w4906:u32)
          n1753 = Bundle By Name(cluster=w4908, "Obs_state"=w4906, "cyclesDone"=w4882, "sequesDone"=w4882) -> (w4905:refnum<class "S4GUI.lvclass">)
        }
        frame 361 {
          # "90: estado de erro."
          # "Timeout= 25s + distancia do target (cada 1000um=1s)"
          # "Espera terminar o movimento do foco do 2ndario para \ndisparar a aquisição do canal."
          n1754 = flat-sequence {
            tunnel: w4954 -> [w4976]
            tunnel: [w4976] -> w4953
            frame #0 {
              n1755 = Tick Count (ms)() -> (millisecond timer value=w4975:u32)
              "time 8" <- w4975
              n1756 = local read "time1"() -> (w4974:u32)
              n1757 = Subtract(x=w4975, y=w4974) -> (x-y=→"delay 78":u32)
            }
          }
          n1758 = call-dynamic "Read TelFocus.lvclass.vi"("error in (no error)"=w4953, "S4GUI in"=w4958) -> ("error out"=w4963:errorcluster, "TelFocus.lvclass"=w4964:refnum<class "TelFocus.lvclass">, "S4GUI out"=w4960:refnum<class "S4GUI.lvclass">)  [unwired: 7 in]
          n1759 = call-dynamic "Read SecMirror.lvclass.vi"("error in (no error)"=w4963, "TelFocus in"=w4964) -> ("error out"=w4932:errorcluster, "SecMirror.lvclass"=w4935:refnum<class "SecMirror.lvclass">, "TelFocus out"=w4962:refnum<class "TelFocus.lvclass">)  [unwired: 7 in]
          n1760 = call-dynamic "Read position.vi"("error in (no error)"=w4932, "SecMirror in"=w4935) -> ("error out"=w4931:errorcluster, "position"=w4928:i32, "SecMirror out"=w4934:refnum<class "SecMirror.lvclass">)  [unwired: 7 in]
          n1761 = call-dynamic "Read target.vi"("error in (no error)"=w4931, "SecMirror in"=w4934) -> ("error out"=w4930:errorcluster, "target"=w4929:i32, "SecMirror out"=w4933:refnum<class "SecMirror.lvclass">)  [unwired: 7 in]
          n1762 = Subtract(x=w4929, y=w4928) -> (x-y=w4927:i32)
          n1763 = Absolute Value(x=w4927) -> (abs(x)=w4926:i32)
          n1764 = call-dynamic "Read State Machine.vi"("error in (no error)"=w4930, "Device in"=w4933) -> ("error out"=w4943:errorcluster, "State Machine.lvclass"=w4946:refnum<class "State Machine.lvclass">, "Device out"=w4956:refnum<class "SecMirror.lvclass">)  [unwired: 7 in]
          n1765 = To Unsigned Long Integer(number=w4926) -> (unsigned 32bit integer=w4923:u32)
          n1766 = Add(x=w4923, y=u32 25000 ("period")) -> (x+y=w4924:u32)
          n1767 = call-dynamic "Verif Clock 2.vi"("error in (no error)"=w4943, "period (ms)"=w4924, "State Machine in"=w4946) -> ("error out"=w4942:errorcluster, "time elapsed"=→"time elapsed 2":u32, "State Machine out"=w4945:refnum<class "State Machine.lvclass">)  [unwired: 6 in]
          n1768 = call-dynamic "Read Timeout 2.vi"("error in (no error)"=w4942, "State Machine in"=w4945) -> ("error out"=w4941:errorcluster, "Timeout 2"=w4919:bool, "State Machine out"=w4944:refnum<class "State Machine.lvclass">)  [unwired: 7 in]
          n1769 = call-dynamic "Read State.vi"("error in (no error)"=w4941, "State Machine in"=w4944) -> ("error out"=w4951:errorcluster, "State"=w4922:i32, "State Machine out"=w4952:refnum<class "State Machine.lvclass">)  [unwired: 7 in]
          n1770 = Equal To 0?(x=w4922) -> (x = 0?=w4917:bool)
          n1771 = Equal?(x=w4922, y=90) -> (x = y?=w4920:bool)
          n1772 = call-dynamic "Write State Machine.vi"("error in (no error)"=w4951, "State Machine.lvclass"=w4952, "Device in"=w4956) -> ("error out"=w4955:errorcluster, "Device out"=w4957:refnum<class "SecMirror.lvclass">)  [unwired: 7 in]
          n1773 = call-dynamic "Write SecMirror.lvclass.vi"("error in (no error)"=w4955, "SecMirror.lvclass"=w4957, "TelFocus in"=w4962) -> ("error out"=w4959:errorcluster, "TelFocus out"=w4961:refnum<class "TelFocus.lvclass">)  [unwired: 7 in]
          n1774 = Or(x=w4920, y=w4919) -> (x .or. y?=w4918:bool)
          n1775 = call-dynamic "Write TelFocus.lvclass.vi"("error in (no error)"=w4959, "TelFocus.lvclass"=w4961, "S4GUI in"=w4960) -> ("error out"=w4948:errorcluster, "S4GUI out"=w4940:refnum<class "S4GUI.lvclass">)  [unwired: 7 in]
          n1776 = case shown="False" w4918 {
            tunnel: w4947 -> [w4967 _]
            tunnel: [w4967 u32 1 ("Obs_state")] -> w4937
            tunnel: w4940 -> [w4966 w4972]
            tunnel: [w4966 w4971] -> w4939
            tunnel: [w4965 FALSE] -> w4916
            tunnel: w4917 -> [w4965 _]
            frame False {
            }
            frame True {
              n1777 = Bundle By Name(cluster=w4972, "Error Msg"="ERROR: moving telescope focus timeout  (S4GUI:HandleObservationSync.vi - state 361)") -> (w4971:refnum<class "S4GUI.lvclass">)
            }
          }
          n1778 = Increment(x=w4937) -> (x+1=w4936:u32)
          n1779 = Select(t=w4936, s=w4916, f=w4937) -> (s? t:f=w4950:u32)
          n1780 = Bundle By Name(cluster=w4939, "Obs_state"=w4950) -> (w4949:refnum<class "S4GUI.lvclass">)
        }
        frame 362 {
          # "Envia dados para o header das imagens (Channel:Run.vi - estado 58)"
          n1781 = call-dynamic "Read AcquisitionA.vi"("error in (no error)"=w5018, "S4ACS_GUI in"=w5019) -> ("error out"=w4995:errorcluster, "Acquisition.lvclass"=w4998:refnum<class "Acquisition.lvclass">, "S4ACS_GUI out"=w5021:refnum<class "S4GUI.lvclass">)  [unwired: 7 in]
          n1782 = call-dynamic "Read enabled.vi"("error in (no error)"=w4995, "Server in"=w4998) -> ("error out"=w4994:errorcluster, "enabled"=w4996:bool, "Server out"=w4997:refnum<class "Acquisition.lvclass">)  [unwired: 7 in]
          n1783 = case shown="True" w4996 {
            tunnel: w4997 -> [w5077 w5092]
            tunnel: w4994 -> [w5076 w5091]
            tunnel: [w5077 w5089] -> w5022
            tunnel: [w5076 w5088] -> w5020
            frame False {
            }
            frame True {
              n1784 = call-dynamic "Read Channel.vi"("error in (no error)"=w5091, "Acquisition in"=w5092) -> ("error out"=w5084:errorcluster, "Channel.lvclass"=w5083:refnum<class "Channel.lvclass">, "Acquisition out"=w5090:refnum<class "Acquisition.lvclass">)  [unwired: 7 in]
              n1785 = call-dynamic "Read State Machine.vi"("error in (no error)"=w5084, "Device in"=w5083) -> ("error out"=w5085:errorcluster, "State Machine.lvclass"=w5087:refnum<class "State Machine.lvclass">, "Device out"=w5081:refnum<class "Channel.lvclass">)  [unwired: 7 in]
              n1786 = call "Next State.vi"("error in (no error)"=w5085, "New_State"=58, "State Machine in"=w5087) -> ("error out"=w5078:errorcluster, "State Machine out"=w5079:refnum<class "State Machine.lvclass">)  [unwired: 7 in]
              n1787 = call-dynamic "Write State Machine.vi"("error in (no error)"=w5078, "State Machine.lvclass"=w5079, "Device in"=w5081) -> ("error out"=w5080:errorcluster, "Device out"=w5082:refnum<class "Channel.lvclass">)  [unwired: 7 in]
              n1788 = call-dynamic "Write Channel.vi"("error in (no error)"=w5080, "Channel.lvclass"=w5082, "Acquisition in"=w5090) -> ("error out"=w5088:errorcluster, "Acquisition out"=w5089:refnum<class "Acquisition.lvclass">)  [unwired: 7 in]
            }
          }
          n1789 = call-dynamic "Write AcquisitionA.vi"("error in (no error)"=w5020, "Acquisition.lvclass"=w5022, "S4ACS_GUI in"=w5021) -> ("error out"=w5013:errorcluster, "S4ACS_GUI out"=w5014:refnum<class "S4GUI.lvclass">)  [unwired: 7 in]
          n1790 = call "Read AcquisitionB.vi"("error in (no error)"=w5013, "S4ACS_GUI in"=w5014) -> ("error out"=w4991:errorcluster, "Acquisition.lvclass"=w4993:refnum<class "Acquisition.lvclass">, "S4ACS_GUI out"=w5011:refnum<class "S4GUI.lvclass">)  [unwired: 7 in]
          n1791 = call-dynamic "Read enabled.vi"("error in (no error)"=w4991, "Server in"=w4993) -> ("error out"=w4990:errorcluster, "enabled"=w4989:bool, "Server out"=w4992:refnum<class "Acquisition.lvclass">)  [unwired: 7 in]
          n1792 = case shown="True" w4989 {
            tunnel: w4992 -> [w5060 w5075]
            tunnel: w4990 -> [w5059 w5074]
            tunnel: [w5060 w5072] -> w5012
            tunnel: [w5059 w5071] -> w5010
            frame False {
            }
            frame True {
              n1793 = call-dynamic "Read Channel.vi"("error in (no error)"=w5074, "Acquisition in"=w5075) -> ("error out"=w5067:errorcluster, "Channel.lvclass"=w5066:refnum<class "Channel.lvclass">, "Acquisition out"=w5073:refnum<class "Acquisition.lvclass">)  [unwired: 7 in]
              n1794 = call-dynamic "Read State Machine.vi"("error in (no error)"=w5067, "Device in"=w5066) -> ("error out"=w5068:errorcluster, "State Machine.lvclass"=w5070:refnum<class "State Machine.lvclass">, "Device out"=w5064:refnum<class "Channel.lvclass">)  [unwired: 7 in]
              n1795 = call "Next State.vi"("error in (no error)"=w5068, "New_State"=58, "State Machine in"=w5070) -> ("error out"=w5061:errorcluster, "State Machine out"=w5062:refnum<class "State Machine.lvclass">)  [unwired: 7 in]
              n1796 = call-dynamic "Write State Machine.vi"("error in (no error)"=w5061, "State Machine.lvclass"=w5062, "Device in"=w5064) -> ("error out"=w5063:errorcluster, "Device out"=w5065:refnum<class "Channel.lvclass">)  [unwired: 7 in]
              n1797 = call-dynamic "Write Channel.vi"("error in (no error)"=w5063, "Channel.lvclass"=w5065, "Acquisition in"=w5073) -> ("error out"=w5071:errorcluster, "Acquisition out"=w5072:refnum<class "Acquisition.lvclass">)  [unwired: 7 in]
            }
          }
          n1798 = call "Write AcquisitionB.vi"("error in (no error)"=w5010, "Acquisition.lvclass"=w5012, "S4ACS_GUI in"=w5011) -> ("error out"=w5006:errorcluster, "S4ACS_GUI out"=w5005:refnum<class "S4GUI.lvclass">)  [unwired: 7 in]
          n1799 = call-dynamic "Read AcquisitionC.vi"("error in (no error)"=w5006, "S4ACS_GUI in"=w5005) -> ("error out"=w4986:errorcluster, "Acquisition.lvclass"=w4988:refnum<class "Acquisition.lvclass">, "S4ACS_GUI out"=w5008:refnum<class "S4GUI.lvclass">)  [unwired: 7 in]
          n1800 = call-dynamic "Read enabled.vi"("error in (no error)"=w4986, "Server in"=w4988) -> ("error out"=w4985:errorcluster, "enabled"=w4984:bool, "Server out"=w4987:refnum<class "Acquisition.lvclass">)  [unwired: 7 in]
          n1801 = case shown="True" w4984 {
            tunnel: [w5042 w5050] -> w5009
            tunnel: [w5043 w5049] -> w5007
            tunnel: w4987 -> [w5043 w5047]
            tunnel: w4985 -> [w5042 w5046]
            frame False {
            }
            frame True {
              n1802 = call-dynamic "Read Channel.vi"("error in (no error)"=w5046, "Acquisition in"=w5047) -> ("error out"=w5054:errorcluster, "Channel.lvclass"=w5055:refnum<class "Channel.lvclass">, "Acquisition out"=w5048:refnum<class "Acquisition.lvclass">)  [unwired: 7 in]
              n1803 = call-dynamic "Read State Machine.vi"("error in (no error)"=w5054, "Device in"=w5055) -> ("error out"=w5053:errorcluster, "State Machine.lvclass"=w5051:refnum<class "State Machine.lvclass">, "Device out"=w5057:refnum<class "Channel.lvclass">)  [unwired: 7 in]
              n1804 = call "Next State.vi"("error in (no error)"=w5053, "New_State"=58, "State Machine in"=w5051) -> ("error out"=w5045:errorcluster, "State Machine out"=w5044:refnum<class "State Machine.lvclass">)  [unwired: 7 in]
              n1805 = call-dynamic "Write State Machine.vi"("error in (no error)"=w5045, "State Machine.lvclass"=w5044, "Device in"=w5057) -> ("error out"=w5058:errorcluster, "Device out"=w5056:refnum<class "Channel.lvclass">)  [unwired: 7 in]
              n1806 = call-dynamic "Write Channel.vi"("error in (no error)"=w5058, "Channel.lvclass"=w5056, "Acquisition in"=w5048) -> ("error out"=w5050:errorcluster, "Acquisition out"=w5049:refnum<class "Acquisition.lvclass">)  [unwired: 7 in]
            }
          }
          n1807 = call-dynamic "Write AcquisitionC.vi"("error in (no error)"=w5009, "Acquisition.lvclass"=w5007, "S4ACS_GUI in"=w5008) -> ("error out"=w5003:errorcluster, "S4ACS_GUI out"=w5002:refnum<class "S4GUI.lvclass">)  [unwired: 7 in]
          n1808 = call-dynamic "Read AcquisitionD.vi"("error in (no error)"=w5003, "S4ACS_GUI in"=w5002) -> ("error out"=w4981:errorcluster, "Acquisition.lvclass"=w4983:refnum<class "Acquisition.lvclass">, "S4ACS_GUI out"=w5001:refnum<class "S4GUI.lvclass">)  [unwired: 7 in]
          n1809 = call-dynamic "Read enabled.vi"("error in (no error)"=w4981, "Server in"=w4983) -> ("error out"=w4980:errorcluster, "enabled"=w4979:bool, "Server out"=w4982:refnum<class "Acquisition.lvclass">)  [unwired: 7 in]
          n1810 = case shown="True" w4979 {
            tunnel: w4980 -> [w5025 w5041]
            tunnel: [w5025 w5040] -> w5004
            tunnel: w4982 -> [w5026 w5031]
            tunnel: [w5026 w5029] -> w5000
            frame False {
            }
            frame True {
              n1811 = call-dynamic "Read Channel.vi"("error in (no error)"=w5041, "Acquisition in"=w5031) -> ("error out"=w5036:errorcluster, "Channel.lvclass"=w5035:refnum<class "Channel.lvclass">, "Acquisition out"=w5030:refnum<class "Acquisition.lvclass">)  [unwired: 7 in]
              n1812 = call-dynamic "Read State Machine.vi"("error in (no error)"=w5036, "Device in"=w5035) -> ("error out"=w5037:errorcluster, "State Machine.lvclass"=w5039:refnum<class "State Machine.lvclass">, "Device out"=w5033:refnum<class "Channel.lvclass">)  [unwired: 7 in]
              n1813 = call "Next State.vi"("error in (no error)"=w5037, "New_State"=58, "State Machine in"=w5039) -> ("error out"=w5027:errorcluster, "State Machine out"=w5028:refnum<class "State Machine.lvclass">)  [unwired: 7 in]
              n1814 = call-dynamic "Write State Machine.vi"("error in (no error)"=w5027, "State Machine.lvclass"=w5028, "Device in"=w5033) -> ("error out"=w5032:errorcluster, "Device out"=w5034:refnum<class "Channel.lvclass">)  [unwired: 7 in]
              n1815 = call-dynamic "Write Channel.vi"("error in (no error)"=w5032, "Channel.lvclass"=w5034, "Acquisition in"=w5030) -> ("error out"=w5040:errorcluster, "Acquisition out"=w5029:refnum<class "Acquisition.lvclass">)  [unwired: 7 in]
            }
          }
          n1816 = call-dynamic "Write AcquisitionD.vi"("error in (no error)"=w5004, "Acquisition.lvclass"=w5000, "S4ACS_GUI in"=w5001) -> ("error out"=w4978:errorcluster, "S4ACS_GUI out"=w4999:refnum<class "S4GUI.lvclass">)  [unwired: 7 in]
          n1817 = flat-sequence {
            tunnel: w4978 -> [w5023]
            tunnel: [w5023] -> w4977
            frame #0 {
              n1818 = Tick Count (ms)() -> (millisecond timer value=→"time9":u32)
            }
          }
